vi "readInFilex.vi"(8 "error in (no error)":errorcluster, 10 "Path":path=path "C:/Users/Administrator/Desktop/Crete/Data/2014/1411/141126/Scripts/Instrument Scripts/Dio64.csv", 11 "AnalogCSVReader in":refnum<class "AnalogCSVReader.lvclass">) -> (0 "error out":errorcluster, 3 "AnalogCSVReader out":refnum<class "AnalogCSVReader.lvclass">)   [LabVIEW 2011, in "AnalogCSVReader.lvclass"]
uses:
  AnalogCSVReader.lvclass
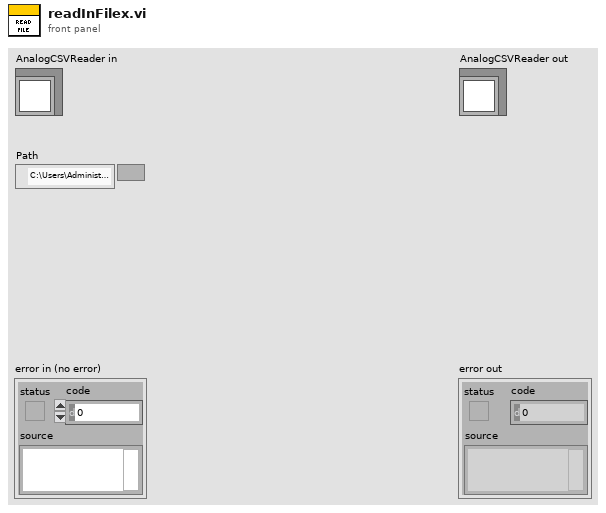
[diagram p1: front panel]
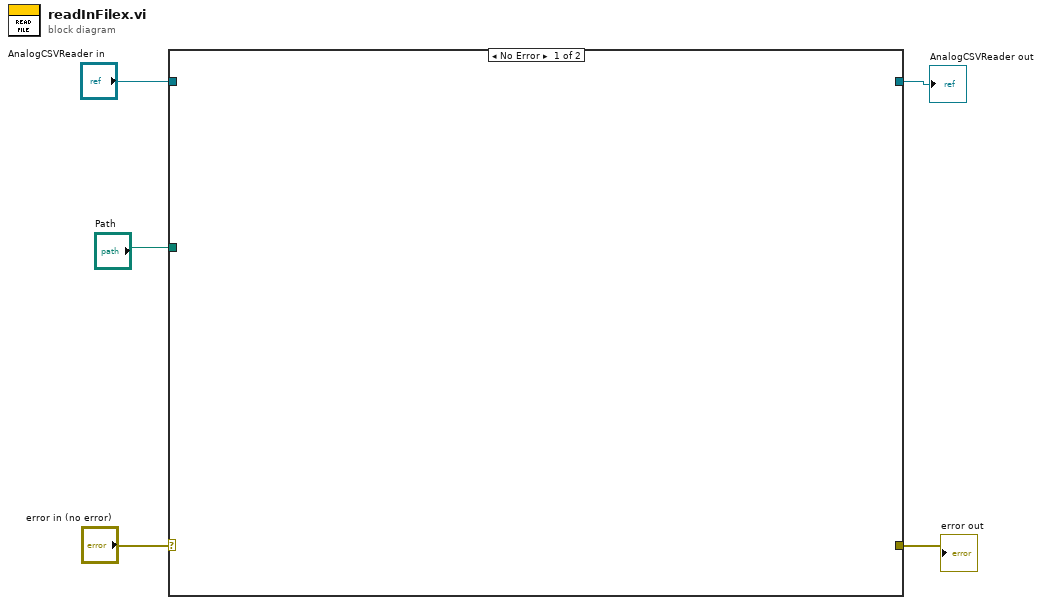
[diagram p0: block diagram]
diagram:
  n1 = case shown="No Error" "error in (no error)" {
    selector: "error in (no error)" -> [w10 w11]
    tunnel: [w7 w12] -> w4
    tunnel: "AnalogCSVReader in" -> [w8 w12]
    tunnel: [w9 w11] -> w2
    tunnel: "Path" -> [w6 _]
    frame No Error {
    }
    frame Error {
    }
  }
  "error out" <- w2
  "AnalogCSVReader out" <- w4
